vi "traj_coe_write.vi"() -> ()   [LabVIEW 2014]
uses:
  <vilib>/Utility/file.llb/Read From Spreadsheet File (DBL).vi
  <vilib>/FPGAPlugInAG/cRIO-9066/niLvFpga_Open_cRIO-9066.vi
  <vilib>/Utility/error.llb/Error Cluster From Error Code.vi
  <vilib>/rvi/errors/niLvFpgaAdjustHostInterfaceError.vi
  <vilib>/rvi/interface/nirviOpenFPGA/nirviOpenFPGA.xnode
  FPGA Bitfiles/forcecontroledu_FPGATarget_EDUreadsub_sPjDGM7eTjE.lvbitx
  FPGA VIs/EDU_read_sub.vi
  <vilib>/rvi/interface/nirviMethod/nirviMethod.xnode
  <vilib>/rvi/errors/niLvFpgaMergeErrorWithErrorCode.vi
  <vilib>/FPGAPlugInAG/cRIO-9066/niLvFpga_StartFifo_cRIO-9066.vi
  <vilib>/FPGAPlugInAG/cRIO-9066/niLvFpga_WriteFifo_cRIO-9066.vi
panel:
  out "writing_done":bool
  in  "stop":bool
  out "qa":dbl[](array[numeric]) format="%.2f"
  out "ta":dbl[](array[numeric]) format="%.2f"
  out "qdda":dbl[](array[numeric])=[0.0, 0.0989990234375, 0.197998046875, 0.2969970703125, 0.396026611328125, 0.495025634765625, 0.594024658203125, 0.693023681640625, 0.79205322265625, 0.89105224609375, 0.99005126953125, 1.089111328125, 1.1881103515625, 1.287109375, 1.3861083984375, 1.485107421875, 1.5841064453125, 1.68310546875, 1.7821044921875, 1.881103515625, 1.9801025390625, 2.0791015625, 2.1781005859375, 2.277099609375, 2.3760986328125, 2.47509765625, 2.5740966796875, 2.673095703125, 2.7720947265625, 2.87109375, 2.9700927734375, 3.0692138671875, 3.168212890625, 3.2672119140625, 3.3662109375, 3.4652099609375, 3.564208984375, 3.6632080078125, 3.76220703125, 3.8612060546875, 3.960205078125, 4.0592041015625, 4.158203125, 4.2572021484375, 4.356201171875, 4.4552001953125, 4.55419921875, 4.6531982421875, 4.752197265625, 4.8511962890625, 4.9501953125, 5.049285888671875, 5.148284912109375, 5.247314453125, 5.3463134765625, 5.4453125, 5.5443115234375, 5.643310546875, 5.7423095703125, 5.84130859375, 5.9403076171875, 6.039306640625, 6.1383056640625, 6.2373046875, 6.3363037109375, 6.435302734375, 6.5343017578125, 6.63330078125, 6.7322998046875, 6.831298828125, 6.9302978515625, 7.029388427734375, 7.128387451171875, 7.227386474609375, 7.326385498046875, 7.4254150390625, 7.5244140625, 7.6234130859375, 7.722412109375, 7.8214111328125, 7.92041015625, 8.0194091796875, 8.118408203125, 8.2174072265625, 8.31640625, 8.4154052734375, 8.514404296875, 8.6134033203125, 8.71240234375, 8.8114013671875, 8.910400390625, 9.009490966796875, 9.108489990234375, 9.207489013671875, 9.306488037109375, 9.405487060546875, 9.504486083984375, 9.603485107421875, 9.7025146484375, 9.801513671875, 9.9005126953125, 9.99951171875, 10.0989990234375, 10.197998046875, 10.2969970703125, 10.39599609375, 10.4949951171875, 10.593994140625, 10.6929931640625, 10.7919921875, 10.8909912109375, 10.989990234375, 11.0889892578125, 11.18798828125, 11.2869873046875, 11.385986328125, 11.4849853515625, 11.584014892578125, 11.683013916015625, 11.782012939453125, 11.881011962890625, 11.980010986328125, 12.079010009765625, 12.178009033203125, 12.277008056640625, 12.376007080078125, 12.475006103515625, 12.574005126953125, 12.673004150390625, 12.772003173828125, 12.871002197265625, 12.970001220703125, 13.069000244140625, 13.167999267578125, 13.266998291015625, 13.365997314453125, 13.464996337890625, 13.563995361328125, 13.662994384765625, 13.761993408203125, 13.860992431640625, 13.959991455078125, 14.058990478515625, 14.157989501953125, 14.256988525390625, 14.355987548828125, 14.454986572265625, 14.553985595703125, 14.65301513671875, 14.75201416015625, 14.85101318359375, 14.95001220703125, 15.04901123046875, 15.14801025390625, 15.24700927734375, 15.34600830078125, 15.44500732421875, 15.54400634765625, 15.64300537109375, 15.74200439453125, 15.84100341796875, 15.94000244140625, 16.03900146484375, 16.13800048828125, 16.23699951171875, 16.33599853515625, 16.43499755859375, 16.53399658203125, 16.63299560546875, 16.73199462890625, 16.83099365234375, 16.92999267578125, 17.02899169921875, 17.12799072265625, 17.22698974609375, 17.32598876953125, 17.42498779296875, 17.52398681640625, 17.62298583984375, 17.72198486328125, 17.821014404296875, 17.920013427734375, 18.019012451171875, 18.118011474609375, 18.217010498046875, 18.316009521484375, 18.415008544921875, 18.514007568359375, 18.613006591796875, 18.712005615234375, 18.811004638671875, 18.910003662109375, 19.009002685546875, 19.108001708984375, 19.207000732421875, 19.305999755859375, 19.404998779296875, 19.503997802734375, 19.602996826171875, 19.701995849609375, 19.800994873046875, 19.899993896484375, 19.998992919921875] format="%.2f"
  out "tba":dbl[](array[numeric]) format="%.2f"
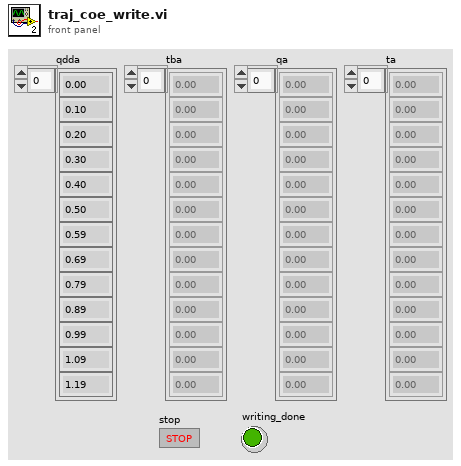
[diagram p1: front panel]
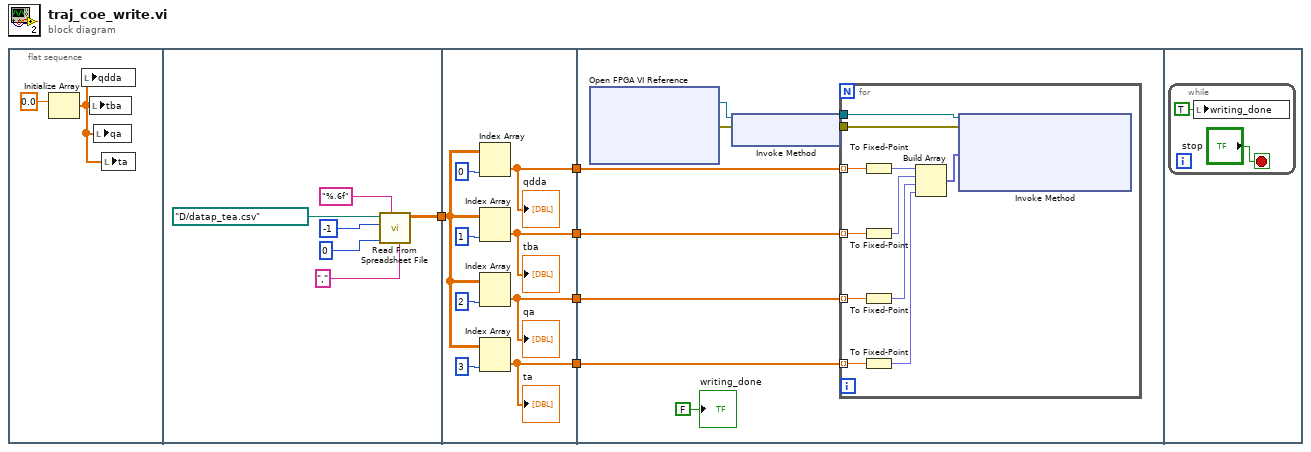
[diagram p0: block diagram]
diagram:
  n1 = flat-sequence {
    tunnel: [w8] -> w5
    tunnel: w5 -> [w18]
    tunnel: [w17] -> w4
    tunnel: [w16] -> w3
    tunnel: [w15] -> w2
    tunnel: [w14] -> w1
    tunnel: w4 -> [w27]
    tunnel: w3 -> [w26]
    tunnel: w2 -> [w25]
    tunnel: w1 -> [w24]
    frame #0 {
      n2 = Initialize Array(0.0 ("element")) -> (w6:dbl[])  [unwired: 1 in]
      n3 = local write "qdda"(w6) -> ()
      n4 = local write "tba"(w6) -> ()
      n5 = local write "qa"(w6) -> ()
      n6 = local write "ta"(w6) -> ()
    }
    frame #1 {
      n7 = call-poly <vilib>:"Read From Spreadsheet File.vi"("delimiter (\\t)"="," ("delimiter (\\t)"), "format (%.3f)"="%.6f" ("format (%d)"), "max characters/row  (no limit:0)"=0, "number of rows (all:-1)"=-1, "file path (dialog if empty)"=path "D:/datap_tea.csv") -> ("all rows"=w8:dbl[][])  [unwired: 2 in, 4 out]
    }
    frame #2 {
      n8 = Index Array(array=w18, index (col)=0 ("disabled index (col)")) -> (element=w17:dbl[])  [unwired: 1 in]
      "qdda" <- w17
      n9 = Index Array(array=w18, index (col)=1 ("disabled index (col)")) -> (element=w16:dbl[])  [unwired: 1 in]
      "tba" <- w16
      n10 = Index Array(array=w18, index (col)=2 ("disabled index (col)")) -> (element=w15:dbl[])  [unwired: 1 in]
      "qa" <- w15
      n11 = Index Array(array=w18, index (col)=3 ("disabled index (col)")) -> (element=w14:dbl[])  [unwired: 1 in]
      "ta" <- w14
    }
    frame #3 {
      n12 = xnode "Open FPGA VI Reference"() -> ("FPGA VI Reference Out"=w31:refnum<k20>, "error out"=w30:errorcluster)  [unwired: 2 in]
      n13 = xnode "Invoke Method"("FPGA VI Reference In"=w31, "error in"=w30) -> ("FPGA VI Reference Out"=w29:refnum<k20>, "error out"=w28:errorcluster)
      n14 = for {
        tunnel: w29 -> [w42]
        tunnel: w28 -> [w41]
        tunnel: w27 -> [w40] mode=indexing
        tunnel: w26 -> [w39] mode=indexing
        tunnel: w25 -> [w38] mode=indexing
        tunnel: w24 -> [w37] mode=indexing
        n15 = To Fixed-Point(number=w40) -> (fixed-point=w36:fxp<+/-,40,15>)  [unwired: 1 in]
        n16 = To Fixed-Point(number=w39) -> (fixed-point=w35:fxp<+/-,40,15>)  [unwired: 1 in]
        n17 = To Fixed-Point(number=w38) -> (fixed-point=w34:fxp<+/-,40,15>)  [unwired: 1 in]
        n18 = To Fixed-Point(number=w37) -> (fixed-point=w33:fxp<+/-,40,15>)  [unwired: 1 in]
        n19 = Build Array(w36, w35, w34, w33) -> (w32:fxp<+/-,40,15>[])
        n20 = xnode "Invoke Method"("FPGA VI Reference In"=w42, "error in"=w41, "Data"=w32) -> ()  [unwired: 1 in, 3 out]
      }
      "writing_done" <- FALSE ("writing_done")
    }
    frame #4 {
      n21 = while {
        stop <- "stop" stop-if-true
        n22 = local write "writing_done"(TRUE ("writing_done")) -> ()
      }
    }
  }
